vi "Launch Replace Window.vi"(8 "error in (no error)":errorcluster, 11 "Main Controller Actor in":refnum<class "Main Controller Actor.lvclass">) -> (0 "error out":errorcluster, 3 "Main Controller Actor out":refnum<class "Main Controller Actor.lvclass">)   [LabVIEW 2015]
uses:
  Main Controller Actor.lvclass
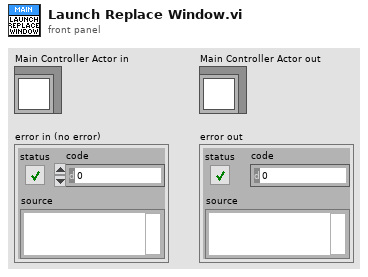
[diagram p1: front panel]
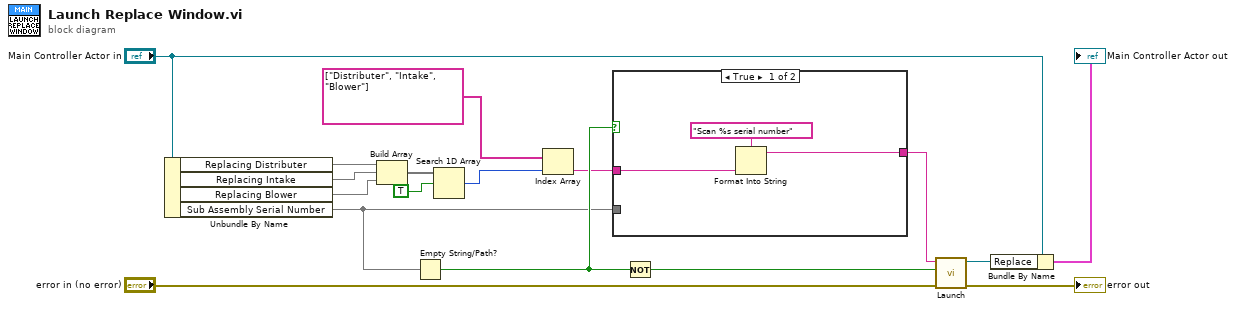
[diagram p0: block diagram]
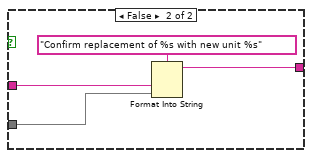
[diagram p2: hidden frame]
diagram:
  n1 = Unbundle By Name("Main Controller Actor in") -> ("Replacing Distributer"=w12, "Replacing Intake"=w11, "Replacing Blower"=w10, "Sub Assembly Serial Number"=w1)
  n2 = Build Array(w12, w11, w10) -> (w9:void[])
  n3 = Empty String/Path?(string/path=w1) -> (empty?=w4:bool)
  n4 = Search 1D Array(1D array=w9, element=TRUE) -> (index of element=w6:i32)  [unwired: 1 in]
  n5 = Index Array(array=string[] ["Distributer", "Intake", "Blower"], index=w6) -> (element=w2:string)
  n6 = case shown="True" w4 {
    tunnel: [w19 w23] -> w3
    tunnel: w2 -> [w18 w22]
    tunnel: w1 -> [_ w21]
    frame True {
      n7 = Format Into String(format string="Scan %s serial number", w18) -> (resulting string=w19:string)  [unwired: 2 in, 1 out]
    }
    frame False {
      n8 = Format Into String(format string="Confirm replacement of %s with new unit %s", w22, w21) -> (resulting string=w23:string)  [unwired: 2 in, 1 out]
    }
  }
  n9 = Not(x=w4) -> (.not. x?=w5:bool)
  n10 = call "Launch.vi"("error in (no error)"="error in (no error)", "OK Visible"=w5, "Message"=w3) -> ("error out"=→"error out":errorcluster, "Actor API out"=w15:refnum<class "Actor API.lvclass">)  [unwired: 7 in]
  n11 = Bundle By Name(cluster="Main Controller Actor in", "Replace"=w15) -> (→"Main Controller Actor out":cluster{})
